vi "Motion Plot sub_VI.vi"(8 "Motion Parameters":T1={"Decel Time (s)"=0.0, "Accel Time (s)"=0.0, "Total Time (s)"=0.0, "Max Accel (mm/s^2)"=0.0, "Max Decel (mm/s^2)"=0.0, "Time step (s)"=0.01} {"Time step (s)" min=0.001}) -> (1 "Acceleration":dbl[](graph), 2 "Velocity":dbl[](graph), 3 "Displacement":dbl[](graph), 4 "V max (mm/s)":dbl, 5 "Dist max (mm)":dbl)   [LabVIEW 2017]
uses:
  <vilib>/imath/engines/lvmath2/RunTimeEngine/BuiltInFunctions/round/NIMS_round(DBL-S).vi
  <vilib>/imath/engines/lvmath2/RunTimeEngine/BuiltInFunctions/zeros/NIMS_V=zeros(I32,I32).vi
  <vilib>/imathl/engines/lvmath/Functions/Error Handling/Create Error.vi
  <vilib>/imath/engines/lvmath2/RunTimeEngine/IndexReplace/NIMS V(S)=S.vi
  <instcachedir>/0/NIMS V(S)=S_3F4D177D41884A9C969E5FA0B22E4B28.lvgen/NIMS V(S)=S_3F4D177D41884A9C969E5FA0B22E4B28_003.vi
  <instcachedir>/0/NIMS V(S)=S_3F4D177D41884A9C969E5FA0B22E4B28.lvgen/NIMS V(S)=S_3F4D177D41884A9C969E5FA0B22E4B28_000.vi
  <vilib>/imath/engines/lvmath2/RunTimeEngine/RangeToken/NIMS_Range_R2 - Float.vi
  <instcachedir>/0/NIMS_Range_R2 - Float_6729C30523D247ACAEE4609355DED762.lvgen/NIMS_Range_R2 - Float_6729C30523D247ACAEE4609355DED762_000.vi
  <vilib>/imath/engines/lvmath2/RunTimeEngine/CommandStatement/MC_CommandStatement_break.vi
  <vilib>/imath/engines/lvmath2/RunTimeSupport/NIMS_Error if Not Equal.vi
  <instcachedir>/0/NIMS_Error if Not Equal_6374CBDCC5AA461FB337545605D07630.lvgen/NIMS_Error if Not Equal_6374CBDCC5AA461FB337545605D07630_000.vi
  <vilib>/imath/engines/lvmath2/RunTimeEngine/ErrorHandling/NIMS_Create Error From Enums.vi
  <vilib>/imath/engines/lvmath2/RunTimeEngine/IndexRead/NIMS V(S).vi
  <instcachedir>/0/NIMS V(S)_0488751826AF41519A22953C041130DC.lvgen/NIMS V(S)_0488751826AF41519A22953C041130DC_000.vi
  <vilib>/imath/engines/lvmath2/RunTimeEngine/NodeEndStatement/NIMS_NodeEndStatement_Output.vi
  <instcachedir>/0/NIMS_NodeEndStatement_Output_53EC0D466D134D7ABD903AC30B43404B.lvgen/NIMS_NodeEndStatement_Output_53EC0D466D134D7ABD903AC30B43404B_005.vi
  <vilib>/imath/engines/lvmath2/RunTimeEngine/ErrorHandling/NIMS_Finalize Error.vi
panel:
  # "Use 0.01s"
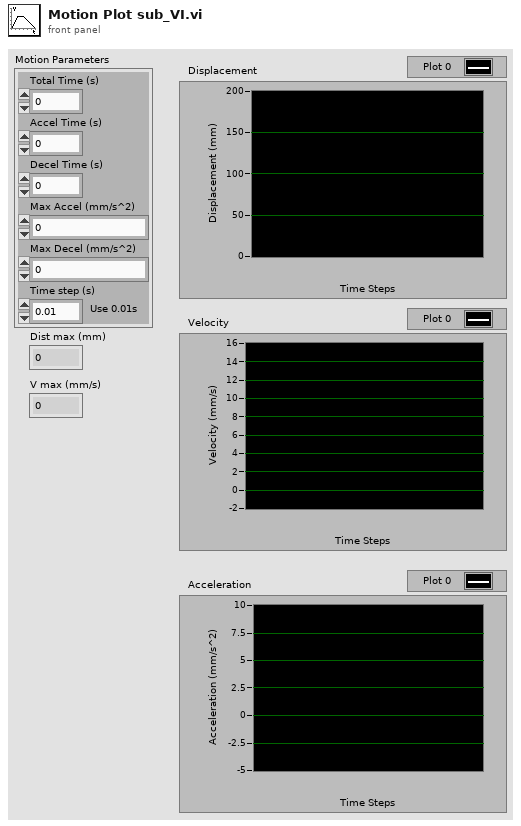
[diagram p1: front panel]
types:
  T1 = cluster{"Decel Time (s)":dbl, "Accel Time (s)":dbl, "Total Time (s)":dbl, "Max Accel (mm/s^2)":dbl, "Max Decel (mm/s^2)":dbl, "Time step (s)":dbl}
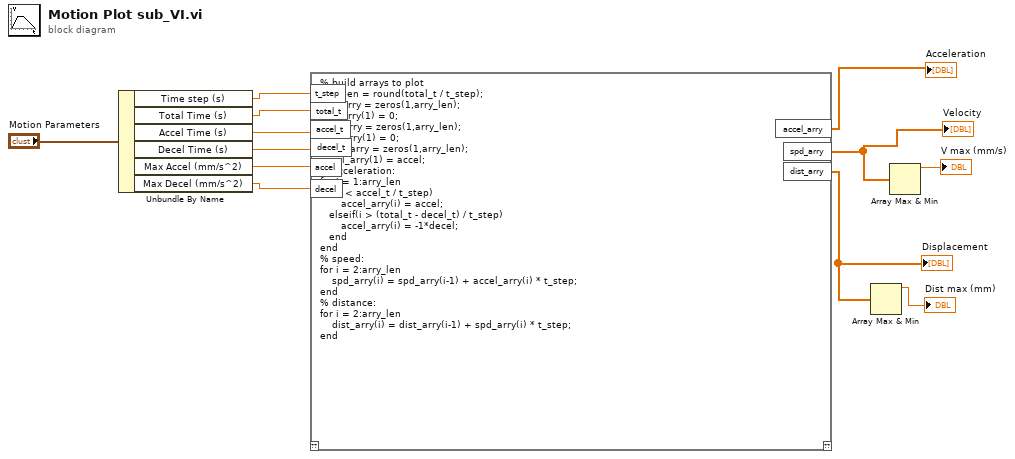
[diagram p0: block diagram]
diagram:
  n1 = Unbundle By Name("Motion Parameters") -> ("Time step (s)"=w6:dbl, "Total Time (s)"=w5:dbl, "Accel Time (s)"=w4:dbl, "Decel Time (s)"=w3:dbl, "Max Accel (mm/s^2)"=w2:dbl, "Max Decel (mm/s^2)"=w1:dbl)
  n2 = mathscript code="% build arrays to plot\narry_len = round(total_t / t_step);\nspd_arry = zeros(1,arry_len);\nspd_arry(1) = 0;\ndist_arry = zeros(1,arry_len);\ndist_arry(1) = 0;\naccel_arry = zeros(1,arry_len);\naccel_arry(1) = accel;\n% acceleration:\nfor i = 1:arry_len\n   if(i < accel_t / t_step)\n       accel_arry(i) = accel;\n   elseif(i > (total_t - decel_t) / t_step)\n       accel_arry(i) = -1*decel;\n   end\nend\n% speed:\nfor i = 2:arry_len\n    spd_arry(i) = spd_arry(i-1) + accel_arry(i) * t_step;\nend\n% distance:\nfor i = 2:arry_len\n    dist_arry(i) = dist_arry(i-1) + spd_arry(i) * t_step;\nend"("total_t"=w5, "t_step"=w6, "accel_t"=w4, "decel_t"=w3, "accel"=w2, "decel"=w1) -> ("accel_arry"=→"Acceleration":dbl[], "spd_arry"=w8:dbl[], "dist_arry"=w7:dbl[])  [unwired: 1 in, 1 out]
  "Velocity" <- w8
  "Displacement" <- w7
  n3 = Array Max & Min(array=w7) -> (max value=→"Dist max (mm)":dbl)  [unwired: 3 out]
  n4 = Array Max & Min(array=w8) -> (max value=→"V max (mm/s)":dbl)  [unwired: 3 out]
